vi "Begin (Trap II).vi"(11 "Image Size":T1=enum."160x120") -> (0 "error out":errorcluster)   [LabVIEW 2012]
doc: "Called before other user functions, this VI is expected to open initial I/O refnums, load in file data, and do all program initialization. Notice that the <B>error out</B> terminal is simply used for data flow. Wiring it to other structures or subVIs ensures that this VI runs first."
uses:
  <vilib>/Rock Robotics/WPI/Camera/WPI_CameraImageSize.ctl
  <vilib>/Rock Robotics/WPI/Camera/WPI_CameraWhite Balance Values.ctl
  <vilib>/Rock Robotics/WPI/Camera/WPI_CameraExposure Values.ctl
  <vilib>/Rock Robotics/WPI/Camera/WPI_CameraFrameRate.ctl
  <vilib>/Rock Robotics/WPI/DriverStation/WPI_DriverStationRobotMode2.ctl
  <vilib>/Rock Robotics/WPI/Joystick/WPI_JoystickDeviceEnum.ctl
  <vilib>/Rock Robotics/SystemInterfaces/Typedef/FPGA_TypedefDigitalModule.ctl
  <vilib>/Rock Robotics/SystemInterfaces/DIO/FPGA_DIOPWMChannel.ctl
  <vilib>/Rock Robotics/SystemInterfaces/DIO/FPGA_DIOChannel.ctl
  <vilib>/Rock Robotics/WPI/Encoder/WPI_EncoderType.ctl
  <vilib>/Rock Robotics/WPI/Solenoid/WPI_SolenoidChannel.ctl
  <vilib>/Rock Robotics/SystemInterfaces/Typedef/FPGA_TypedefSolenoidModule.ctl
  <vilib>/Rock Robotics/WPI/Solenoid/WPI_SolenoidValue.ctl
  <vilib>/Rock Robotics/WPI/SafetyOutput/WPI_SafetyOutputConfigMenu.ctl
  <vilib>/Rock Robotics/SystemInterfaces/DIO/FPGA_DIORelayChannel.ctl
  <vilib>/Rock Robotics/SystemInterfaces/Typedef/FPGA_TypedefAnalogModuleForGyro.ctl
  <vilib>/Rock Robotics/SystemInterfaces/AI/FPGA_AIGyroChannel.ctl
  Robot Global Data.vi
  <vilib>/Rock Robotics/WPI/MotorControl/WPI_MotorControlOpen Jaguar.vi
  <vilib>/Rock Robotics/WPI/Counter/WPI_CounterDigitalInputToDigitalSource.vi
  <vilib>/Rock Robotics/WPI/Solenoid/WPI_SolenoidOpenSingle.vi
  <vilib>/Rock Robotics/WPI/Solenoid/WPI_SolenoidSetEnum.vi
  <vilib>/Rock Robotics/WPI/RobotDrive/WPI_RobotDriveOpen2MotorWithJaguar.vi
  <vilib>/Rock Robotics/WPI/Solenoid/WPI_SolenoidOpenDouble.vi
  <vilib>/Rock Robotics/WPI/Compressor/WPI_CompressorGetSetRefNum.vi
  <vilib>/Rock Robotics/WPI/RobotDrive/WPI_RobotDriveOpen4MotorWithTalon.vi
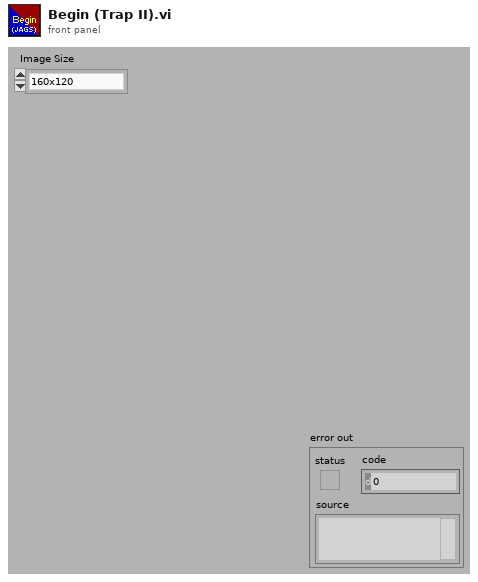
[diagram p1: front panel]
types:
  T1 = typedef "WPI_CameraImageSize.ctl" = enum16{"640x480", "320x240", "160x120"}
  T2 = typedef "FPGA_AIGyroChannel.ctl" = enum8{"AI 1", "AI 2", "Invalid"}
  T3 = typedef "FPGA_TypedefAnalogModuleForGyro.ctl" = enum16{"Analog Module 1"}
  T4 = typedef "WPI_SolenoidChannel.ctl" = enum8{"Solenoid 1", "Solenoid 2", "Solenoid 3", "Solenoid 4", "Solenoid 5", "Solenoid 6", "Solenoid 7", "Solenoid 8", "Invalid"}
  T5 = typedef "WPI_SolenoidValue.ctl" = enum16{"Off", "On", "Forward", "Reverse"}
  T6 = typedef "FPGA_DIOChannel.ctl" = enum8{"DIO 1", "DIO 2", "DIO 3", "DIO 4", "DIO 5", "DIO 6", "DIO 7", "DIO 8", "DIO 9", "DIO 10", "DIO 11", "DIO 12", "DIO 13", "DIO 14", "Invalid"}
  T7 = typedef "FPGA_DIORelayChannel.ctl" = enum8{"Relay 1", "Relay 2", "Relay 3", "Relay 4", "Relay 5", "Relay 6", "Relay 7", "Relay 8", "Invalid"}
  T8 = typedef "FPGA_TypedefDigitalModule.ctl" = enum16{"Digital Module 1", "Digital Module 2"}
  T9 = typedef "WPI_SafetyOutputConfigMenu.ctl" = enum16{"Enable", "Disable"}
  T10 = typedef "FPGA_DIOPWMChannel.ctl" = enum8{"PWM 1", "PWM 2", "PWM 3", "PWM 4", "PWM 5", "PWM 6", "PWM 7", "PWM 8", "PWM 9", "PWM 10", "Invalid"}
  T11 = typedef "WPI_EncoderType.ctl" = enum16{"1x", "2x", "4x"}
  T12 = typedef "FPGA_TypedefSolenoidModule.ctl" = enum16{"Solenoid Module 1", "Solenoid Module 2"}
  T13 = typedef "WPI_JoystickDeviceEnum.ctl" = enum16{"USB 1", "USB 2", "USB 3", "USB 4", "Kinect 1", "Kinect 2"}
  T14 = typedef "WPI_DriverStationRobotMode2.ctl" = enum16{"Autonomous Disabled", "Autonomous Enabled", "Teleop Disabled", "Teleop Enabled", "Timeout", "Finish", "Test Disabled", "Test Enabled"}
  T15 = typedef "WPI_CameraFrameRate.ctl" = u32
  T16 = typedef "WPI_CameraExposure Values.ctl" = enum16{"Auto", "Flicker-free 50 Hz", "Flicker-free 60 Hz", "Hold current"}
  T17 = typedef "WPI_CameraWhite Balance Values.ctl" = enum16{"Auto", "Fixed indoor", "Fixed outdoor 1", "Fixed outdoor 2", "Fixed fluorescent 1", "Fixed fluorescent 2", "Hold current"}
  T18 = typedef "WPI_RobotDriveDevRef.ctl" = cluster{"DevStatus":errorcluster, "Motors[]":T19[], "Square Inputs":bool, "Max Output":dbl, "Isochronous":bool}
  T19 = typedef "WPI_MotorControlDeviceRef.ctl" = cluster{"DeviceStatus":errorcluster, "Type":enum16{"PWM", "CAN"}, "PWM":cluster{"Digital Module":T8, "PWM Channel":T10, "DeadBand":T20}, "CAN":cluster{"Device Number":u8, "Control Mode":T21, "Semaphore":T22, "Max Vout":dbl}, "Invert":bool, "TransformRef":T23, "InvTransformRef":T23}
  T20 = typedef "WPI_PWMDeadband.ctl" = cluster{"Name":string, "maxPositivePwm":i32, "minPositivePwm":i32, "centerPwm":i32, "maxNegativePwm":i32, "minNegativePwm":i32, "angularRange":u16}
  T21 = typedef "WPI_CANJaguar_ControlMode.ctl" = enum8{"Percent VBus", "Current", "Speed", "Position", "Voltage"}
  T22 = typedef "Semaphore RefNum" = refnum<k1>
  T23 = typedef "WPI_PWMTransform_ConPane.ctl" = refnum<vi>
  T24 = typedef "WPI_DigitalInputDevRef.ctl" = cluster{"DevStatus":errorcluster, "DIO Channel":T6, "Digital Module":T8}
  T25 = typedef "FPGA_CounterEncoderSourceConvertionLVSourceType.ctl" = cluster{"DevStatus":errorcluster, "AnalogTriggerMode?":bool, "DigitalMode":cluster{"Digital Module":T8, "DIO Channel":T26}, "AnalogTriggerMode":cluster{"AnalogTriggerIndex":T27, "OutputType":T28}}
  T26 = typedef "FPGA_DIODigitalSourceChannel.ctl" = enum8{"DIO 1", "DIO 2", "DIO 3", "DIO 4", "DIO 5", "DIO 6", "DIO 7", "DIO 8", "DIO 9", "DIO 10", "DIO 11", "DIO 12", "DIO 13", "DIO 14", "Disabled"}
  T27 = typedef "FPGA_AnalogTriggerIndex.ctl" = enum8{"Trig 0", "Trig 1", "Trig 2", "Trig 3", "Trig 4", "Trig 5", "Trig 6", "Trig 7", "Invalid"}
  T28 = typedef "FPGA_AnalogTriggerOutType.ctl" = enum16{"InWindow", "TriggerState", "Rising", "Falling"}
  T29 = typedef "WPI_CameraDevRef.ctl" = cluster{"Camera Address":string, "CameraStatus":errorcluster, "Acquire Image Notifier":refnum<notifier>}
  T30 = typedef "WPI_JoystickDevRef.ctl" = cluster{"Device":T13}
  T31 = typedef "WPI_EncoderDevRef.ctl" = cluster{"DevStatus":errorcluster, "EncoderIndex":T32, "CounterIndex":T33, "DistancePerCount":dbl, "Decoding Type":T11}
  T32 = typedef "FPGA_EncoderIdx.ctl" = enum8{"Enc 0", "Enc 1", "Enc 2", "Enc 3", "Invalid"}
  T33 = typedef "FPGA_CounterCtrSystemIndex.ctl" = enum8{"Ctr 0", "Ctr 1", "Ctr 2", "Ctr 3", "Ctr 4", "Ctr 5", "Ctr 6", "Ctr 7", "Invalid"}
  T34 = typedef "WPI_DigitalOutputDevRef.ctl" = cluster{"Digital Module":T8, "DIO Channel":T6, "DevStatus":errorcluster}
  T35 = typedef "WPI_SolenoidDevRef.ctl" = cluster{"DevStatus":errorcluster, "Solenoid Module":T12, "Forward Solenoid Channel":T4, "Reverse Solenoid Channel":T4}
  T36 = typedef "WPI_GyroDevRef.ctl" = cluster{"DevStatus":errorcluster, "Analog Module":T37, "Analog Channel":T38, "Offset":dbl, "Gain (VoltsPerDegree/Second)":dbl}
  T37 = typedef "FPGA_TypedefAnalogModule.ctl" = enum16{"Analog Module 1", "Analog Module 2"}
  T38 = typedef "FPGA_AIChannel.ctl" = enum8{"AI 1", "AI 2", "AI 3", "AI 4", "AI 5", "AI 6", "AI 7", "AI 8", "Invalid"}
  T39 = typedef "WPI_CompressorDevRef.ctl" = cluster{"DevStatus":errorcluster, "DigitalInputDevRef":T24, "RelayDevRef":T40}
  T40 = typedef "WPI_RelayDevRef.ctl" = cluster{"DevStatus":errorcluster, "Relay Channel":T7, "Digital Module":T8, "Relay Direction":T41}
  T41 = typedef "WPI_RelayDirection.ctl" = enum16{"Both directions", "Forward only", "Reverse only"}
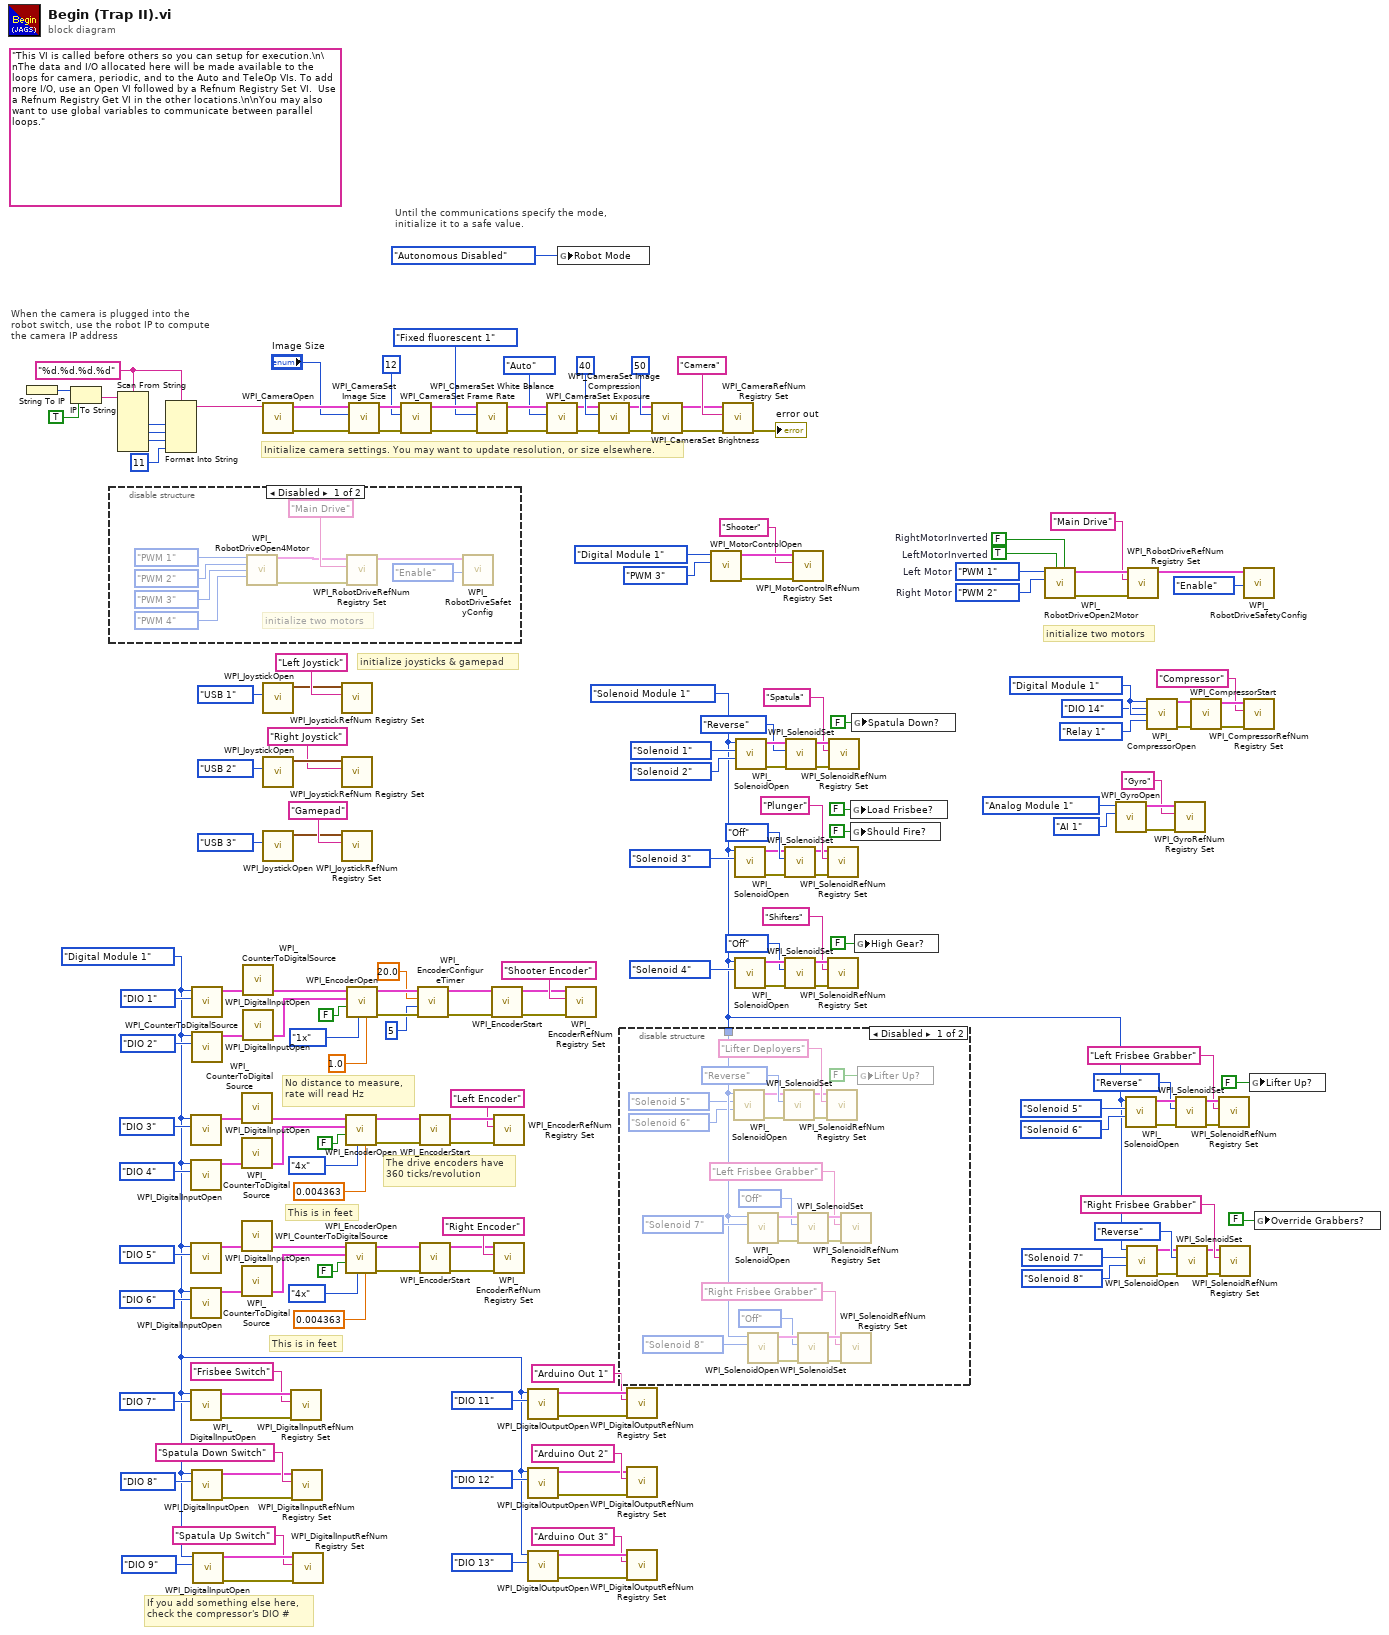
[diagram p0: block diagram]
diagram:
  w53 = FPGA_TypedefDigitalModule."Digital Module 1" ("Pressure Switch Digital Module (Module 1)")
  w77 = FPGA_DIOPWMChannel."PWM 2"  # Right Motor
  w78 = FPGA_DIOPWMChannel."PWM 1"  # Left Motor
  w82 = TRUE  # LeftMotorInverted
  w83 = FALSE  # RightMotorInverted
  w7 = FPGA_TypedefSolenoidModule."Solenoid Module 1" ("Solenoid Module (Module 1)")
  w25 = FPGA_TypedefDigitalModule."Digital Module 1" ("Digital Module (Module 1)")
  w156 = "%d.%d.%d.%d" ("format string")
  (unwired) "This VI is called before others so you can setup for execution.\n\nThe data and I/O allocated here will be made available to the loops for camera, periodic, and to the Auto and TeleOp VIs. To add more I/O, use an Open VI followed by a Refnum Registry Set VI.  Use a Refnum Registry Get VI in the other locations.\n\nYou may also want to use global variables to communicate between parallel loops."
  # "If you add something else here,\ncheck the compressor's DIO #"
  # "No distance to measure,\nrate will read Hz"
  # "The drive encoders have\n360 ticks/revolution"
  # "This is in feet"
  # "This is in feet"
  # "initialize two motors"
  # "initialize joysticks & gamepad"
  # "Until the communications specify the mode,\ninitialize it to a safe value."
  # "When the camera is plugged into the\nrobot switch, use the robot IP to compute\nthe camera IP address"
  # "Initialize camera settings. You may want to update resolution, or size elsewhere."
  n1 = String To IP() -> (0:w163:u32)  [unwired: 1 in]
  n2 = IP To String(1:TRUE ("dot notation? (F)"), 2:w163) -> (0:w161:string)
  n3 = disable-structure shown="Disabled" {
    frame Disabled {
      # "initialize two motors"
      n4 = call-poly <vilib>:"WPI_RobotDriveOpen4Motor.vi"("Rear Left Motor"=FPGA_DIOPWMChannel."PWM 1", "Rear Right Motor"=FPGA_DIOPWMChannel."PWM 2" ("Rear Left Motor"), "Front Left Motor"=FPGA_DIOPWMChannel."PWM 3" ("Rear Left Motor"), "Front Right Motor"=FPGA_DIOPWMChannel."PWM 4" ("Rear Left Motor")) -> ("RobotDriveDevRef"=w190:T18, "error out"=w189:errorcluster)  [unwired: 10 in]
      n5 = call <vilib>:"WPI_RobotDriveRefNum Registry Set.vi"("error in (no error)"=w189, "refnum name"="Main Drive", "RobotDriveDevRef"=w190) -> ("RobotDriveDevRef"=w192:T18)  [unwired: 8 out]
      n6 = call <vilib>:"WPI_RobotDriveSafetyConfig.vi"("mode"=WPI_SafetyOutputConfigMenu."Enable", "RobotDriveDevRef"=w192) -> ()  [unwired: 8 in, 2 out]
    }
    frame Enabled {
    }
  }
  n7 = Scan From String(format string=w156, input string=w161) -> (output 1=w160:i32, output 2=w159:i32, output 3=w158:i32)  [unwired: 7 in, 3 out]
  n8 = Format Into String(format string=w156, w160, w159, w158, 11 ("Compression")) -> (resulting string=w154:string)  [unwired: 2 in, 1 out]
  n9 = call <vilib>:"WPI_DigitalInputOpen.vi"("DIO Channel"=FPGA_DIOChannel."DIO 3" ("CS Channel"), "Digital Module (Module 1)"=w25) -> ("DigitalInputDevRef"=w105:T24)  [unwired: 1 in, 8 out]
  n10 = call <vilib>:"WPI_DigitalInputOpen.vi"("DIO Channel"=FPGA_DIOChannel."DIO 4" ("Clock Channel"), "Digital Module (Module 1)"=w25) -> ("DigitalInputDevRef"=w106:T24)  [unwired: 1 in, 8 out]
  n11 = call <vilib>:"WPI_DigitalInputOpen.vi"("DIO Channel"=FPGA_DIOChannel."DIO 5" ("CS Channel"), "Digital Module (Module 1)"=w25) -> ("DigitalInputDevRef"=w90:T24)  [unwired: 1 in, 8 out]
  n12 = call <vilib>:"WPI_DigitalInputOpen.vi"("DIO Channel"=FPGA_DIOChannel."DIO 6" ("Clock Channel"), "Digital Module (Module 1)"=w25) -> ("DigitalInputDevRef"=w89:T24)  [unwired: 1 in, 8 out]
  n13 = call <vilib>:"WPI_DigitalInputOpen.vi"("DIO Channel"=FPGA_DIOChannel."DIO 7", "Digital Module (Module 1)"=w25) -> ("error out"=w55:errorcluster, "DigitalInputDevRef"=w56:T24)  [unwired: 8 in]
  n14 = call <vilib>:"WPI_DigitalInputOpen.vi"("DIO Channel"=FPGA_DIOChannel."DIO 1" ("CS Channel"), "Digital Module (Module 1)"=w25) -> ("DigitalInputDevRef"=w131:T24)  [unwired: 1 in, 8 out]
  n15 = call <vilib>:"WPI_DigitalInputOpen.vi"("DIO Channel"=FPGA_DIOChannel."DIO 2" ("Clock Channel"), "Digital Module (Module 1)"=w25) -> ("DigitalInputDevRef"=w130:T24)  [unwired: 1 in, 8 out]
  n16 = call <vilib>:"WPI_DigitalInputOpen.vi"("DIO Channel"=FPGA_DIOChannel."DIO 8", "Digital Module (Module 1)"=w25) -> ("error out"=w44:errorcluster, "DigitalInputDevRef"=w43:T24)  [unwired: 8 in]
  n17 = call <vilib>:"WPI_DigitalInputOpen.vi"("DIO Channel"=FPGA_DIOChannel."DIO 9", "Digital Module (Module 1)"=w25) -> ("error out"=w39:errorcluster, "DigitalInputDevRef"=w40:T24)  [unwired: 8 in]
  n18 = call-poly <vilib>:"WPI_CounterToDigitalSource.vi"("DigitalInputDevRef"=w105) -> ("Digital Source"=w102:T25)  [unwired: 6 out]
  n19 = call-poly <vilib>:"WPI_CounterToDigitalSource.vi"("DigitalInputDevRef"=w106) -> ("Digital Source"=w103:T25)  [unwired: 6 out]
  n20 = call-poly <vilib>:"WPI_CounterToDigitalSource.vi"("DigitalInputDevRef"=w90) -> ("Digital Source"=w93:T25)  [unwired: 6 out]
  n21 = call-poly <vilib>:"WPI_CounterToDigitalSource.vi"("DigitalInputDevRef"=w89) -> ("Digital Source"=w92:T25)  [unwired: 6 out]
  n22 = call-poly <vilib>:"WPI_CounterToDigitalSource.vi"("DigitalInputDevRef"=w131) -> ("Digital Source"=w134:T25)  [unwired: 6 out]
  n23 = call-poly <vilib>:"WPI_CounterToDigitalSource.vi"("DigitalInputDevRef"=w130) -> ("Digital Source"=w133:T25)  [unwired: 6 out]
  n24 = call <vilib>:"WPI_CameraOpen.vi"("Camera Address"=w154) -> ("error out"=w175:errorcluster, "CameraDevRef"=w176:T29)  [unwired: 1 in, 8 out]
  n25 = call <vilib>:"WPI_JoystickOpen.vi"("JoystickDevice"=WPI_JoystickDeviceEnum."USB 1") -> ("JoystickDevRef"=w152:T30)  [unwired: 10 in]
  n26 = call <vilib>:"WPI_JoystickOpen.vi"("JoystickDevice"=WPI_JoystickDeviceEnum."USB 2") -> ("JoystickDevRef"=w148:T30)  [unwired: 10 in]
  n27 = call <vilib>:"WPI_JoystickOpen.vi"("JoystickDevice"=WPI_JoystickDeviceEnum."USB 3") -> ("JoystickDevRef"=w145:T30)  [unwired: 10 in]
  n28 = call <vilib>:"WPI_DigitalInputRefNum Registry Set.vi"("error in (no error)"=w55, "refnum name"="Frisbee Switch", "DigitalInputDevRef"=w56) -> ()  [unwired: 7 in, 2 out]
  n29 = call <vilib>:"WPI_DigitalInputRefNum Registry Set.vi"("error in (no error)"=w44, "refnum name"="Spatula Down Switch", "DigitalInputDevRef"=w43) -> ()  [unwired: 7 in, 2 out]
  n30 = call <vilib>:"WPI_DigitalInputRefNum Registry Set.vi"("error in (no error)"=w39, "refnum name"="Spatula Up Switch", "DigitalInputDevRef"=w40) -> ()  [unwired: 7 in, 2 out]
  n31 = call <vilib>:"WPI_JoystickRefNum Registry Set.vi"("refnum name"="Left Joystick", "JoystickDevRef"=w152) -> ()  [unwired: 8 in, 2 out]
  n32 = call <vilib>:"WPI_JoystickRefNum Registry Set.vi"("refnum name"="Right Joystick", "JoystickDevRef"=w148) -> ()  [unwired: 8 in, 2 out]
  n33 = call <vilib>:"WPI_JoystickRefNum Registry Set.vi"("refnum name"="Gamepad", "JoystickDevRef"=w145) -> ()  [unwired: 8 in, 2 out]
  n34 = call <vilib>:"WPI_EncoderOpen.vi"("DistancePerCount"=0.004363, "Decoding Type"=WPI_EncoderType."4x", "Invert Direction (False)"=FALSE, "BSource"=w103, "ASource"=w102) -> ("error out"=w108:errorcluster, "EncoderDevRef"=w107:T31)  [unwired: 5 in]
  n35 = call <vilib>:"WPI_EncoderOpen.vi"("DistancePerCount"=0.004363, "Decoding Type"=WPI_EncoderType."4x", "Invert Direction (False)"=FALSE, "BSource"=w92, "ASource"=w93) -> ("error out"=w87:errorcluster, "EncoderDevRef"=w88:T31)  [unwired: 5 in]
  n36 = call <vilib>:"WPI_EncoderOpen.vi"("DistancePerCount"=1.0, "Decoding Type"=WPI_EncoderType."1x", "Invert Direction (False)"=FALSE, "BSource"=w133, "ASource"=w134) -> ("error out"=w63:errorcluster, "EncoderDevRef"=w64:T31)  [unwired: 5 in]
  n37 = call <vilib>:"WPI_CameraSet Image Size.vi"("error in (no error)"=w175, "Image Size"="Image Size", "CameraDevRef"=w176) -> ("error out"=w174:errorcluster, "CameraDevRef Out"=w177:T29)  [unwired: 7 out]
  n38 = call <vilib>:"WPI_CameraSet Frame Rate.vi"("error in (no error)"=w174, "Frame Rate (fps)"=T15 12, "CameraDevRef"=w177) -> ("error out"=w173:errorcluster, "CameraDevRef Out"=w179:T29)  [unwired: 7 out]
  n39 = call <vilib>:"WPI_EncoderConfigureTimer.vi"("error in (no error)"=w63, "Number Samples to Average"=u8 5, "Minimum Rate"=20.0, "EncoderDevRef"=w64) -> ("error out"=w62:errorcluster, "EncoderDevRef"=w61:T31)  [unwired: 6 in]
  n40 = call <vilib>:"WPI_EncoderStart.vi"("error in (no error)"=w108, "EncoderDevRef"=w107) -> ("error out"=w109:errorcluster, "EncoderDevRef"=w110:T31)  [unwired: 8 in]
  n41 = call <vilib>:"WPI_EncoderStart.vi"("error in (no error)"=w87, "EncoderDevRef"=w88) -> ("error out"=w86:errorcluster, "EncoderDevRef"=w85:T31)  [unwired: 8 in]
  n42 = call <vilib>:"WPI_CameraSet White Balance.vi"("error in (no error)"=w173, "White Balance"=WPI_CameraWhite_Balance_Values."Fixed fluorescent 1", "CameraDevRef"=w179) -> ("error out"=w172:errorcluster, "CameraDevRef Out"=w178:T29)  [unwired: 7 out]
  n43 = call <vilib>:"WPI_EncoderStart.vi"("error in (no error)"=w62, "EncoderDevRef"=w61) -> ("error out"=w129:errorcluster, "EncoderDevRef"=w128:T31)  [unwired: 8 in]
  n44 = call <vilib>:"WPI_EncoderRefNum Registry Set.vi"("error in (no error)"=w109, "refnum name"="Left Encoder", "EncoderDevRef"=w110) -> ()  [unwired: 7 in, 2 out]
  n45 = call <vilib>:"WPI_EncoderRefNum Registry Set.vi"("error in (no error)"=w86, "refnum name"="Right Encoder", "EncoderDevRef"=w85) -> ()  [unwired: 7 in, 2 out]
  n46 = call <vilib>:"WPI_DigitalOutputOpen.vi"("DIO Channel"=FPGA_DIOChannel."DIO 11", "Digital Module (Module 1)"=w25) -> ("error out"=w35:errorcluster, "DigitalOutputDevRef"=w36:T34)  [unwired: 8 in]
  n47 = call <vilib>:"WPI_DigitalOutputOpen.vi"("DIO Channel"=FPGA_DIOChannel."DIO 12", "Digital Module (Module 1)"=w25) -> ("error out"=w32:errorcluster, "DigitalOutputDevRef"=w31:T34)  [unwired: 8 in]
  n48 = call <vilib>:"WPI_DigitalOutputOpen.vi"("DIO Channel"=FPGA_DIOChannel."DIO 13", "Digital Module (Module 1)"=w25) -> ("error out"=w27:errorcluster, "DigitalOutputDevRef"=w28:T34)  [unwired: 8 in]
  n49 = call <vilib>:"WPI_CameraSet Exposure.vi"("error in (no error)"=w172, "Exposure"=WPI_CameraExposure_Values."Auto", "CameraDevRef"=w178) -> ("error out"=w171:errorcluster, "CameraDevRef Out"=w181:T29)  [unwired: 7 out]
  n50 = global write "Robot Global Data.vi" "Robot Mode"(WPI_DriverStationRobotMode2."Autonomous Disabled" ("Robot Mode")) -> ()
  n51 = call <vilib>:"WPI_EncoderRefNum Registry Set.vi"("error in (no error)"=w129, "refnum name"="Shooter Encoder", "EncoderDevRef"=w128) -> ()  [unwired: 7 in, 2 out]
  n52 = call <vilib>:"WPI_CameraSet Image Compression.vi"("error in (no error)"=w171, "Compression"=40, "CameraDevRef"=w181) -> ("error out"=w170:errorcluster, "CameraDevRef Out"=w180:T29)  [unwired: 7 out]
  n53 = disable-structure shown="Disabled" {
    disable-tunnel: w7 -> [w205 _]
    frame Disabled {
      n54 = call-poly <vilib>:"WPI_SolenoidOpen.vi"("Reverse Solenoid Channel"=WPI_SolenoidChannel."Solenoid 6", "Forward Solenoid Channel"=WPI_SolenoidChannel."Solenoid 5" ("Solenoid Channel"), "Solenoid Module (Module 1)"=w205) -> ("error out"=w198:errorcluster, "SolenoidDevRef"=w197:T35)  [unwired: 7 in]
      n55 = call-poly <vilib>:"WPI_SolenoidOpen.vi"("Solenoid Channel"=WPI_SolenoidChannel."Solenoid 7", "Solenoid Module (Module 1)"=w205) -> ("error out"=w215:errorcluster, "SolenoidDevRef"=w214:T35)  [unwired: 8 in]
      n56 = call-poly <vilib>:"WPI_SolenoidOpen.vi"("Solenoid Channel"=WPI_SolenoidChannel."Solenoid 8", "Solenoid Module (Module 1)"=w205) -> ("error out"=w210:errorcluster, "SolenoidDevRef"=w211:T35)  [unwired: 8 in]
      n57 = call-poly <vilib>:"WPI_SolenoidSet.vi"("error in (no error)"=w198, "Value"=WPI_SolenoidValue."Reverse", "SolenoidDevRef"=w197) -> ("error out"=w199:errorcluster, "SolenoidDevRef"=w200:T35)  [unwired: 7 in]
      n58 = call-poly <vilib>:"WPI_SolenoidSet.vi"("error in (no error)"=w215, "Value"=WPI_SolenoidValue."Off", "SolenoidDevRef"=w214) -> ("error out"=w216:errorcluster, "SolenoidDevRef"=w217:T35)  [unwired: 7 in]
      n59 = call-poly <vilib>:"WPI_SolenoidSet.vi"("error in (no error)"=w210, "Value"=WPI_SolenoidValue."Off", "SolenoidDevRef"=w211) -> ("error out"=w209:errorcluster, "SolenoidDevRef"=w208:T35)  [unwired: 7 in]
      n60 = call <vilib>:"WPI_SolenoidRefNum Registry Set.vi"("error in (no error)"=w199, "refnum name"="Lifter Deployers", "SolenoidDevRef"=w200) -> ()  [unwired: 7 in, 2 out]
      n61 = call <vilib>:"WPI_SolenoidRefNum Registry Set.vi"("error in (no error)"=w216, "refnum name"="Left Frisbee Grabber", "SolenoidDevRef"=w217) -> ()  [unwired: 7 in, 2 out]
      n62 = call <vilib>:"WPI_SolenoidRefNum Registry Set.vi"("error in (no error)"=w209, "refnum name"="Right Frisbee Grabber", "SolenoidDevRef"=w208) -> ()  [unwired: 7 in, 2 out]
      n63 = global write "Robot Global Data.vi" "Lifter Up?"(FALSE ("High Gear?")) -> ()
    }
    frame Enabled {
    }
  }
  n64 = call <vilib>:"WPI_DigitalOutputRefNum Registry Set.vi"("error in (no error)"=w35, "refnum name"="Arduino Out 1", "DigitalOutputDevRef"=w36) -> ()  [unwired: 7 in, 2 out]
  n65 = call <vilib>:"WPI_DigitalOutputRefNum Registry Set.vi"("error in (no error)"=w32, "refnum name"="Arduino Out 2", "DigitalOutputDevRef"=w31) -> ()  [unwired: 7 in, 2 out]
  n66 = call <vilib>:"WPI_DigitalOutputRefNum Registry Set.vi"("error in (no error)"=w27, "refnum name"="Arduino Out 3", "DigitalOutputDevRef"=w28) -> ()  [unwired: 7 in, 2 out]
  n67 = call <vilib>:"WPI_CameraSet Brightness.vi"("error in (no error)"=w170, "Brightness"=50, "CameraDevRef"=w180) -> ("error out"=w168:errorcluster, "CameraDevRef Out"=w169:T29)  [unwired: 7 out]
  n68 = call-poly <vilib>:"WPI_MotorControlOpen.vi"("PWM Channel"=FPGA_DIOPWMChannel."PWM 3", "Digital Module (Module 1)"=FPGA_TypedefDigitalModule."Digital Module 1") -> ("error out"=w140:errorcluster, "MotorControlDeviceRef"=w141:T19)  [unwired: 8 in]
  n69 = call <vilib>:"WPI_CameraRefNum Registry Set.vi"("error in (no error)"=w168, "refnum name"="Camera", "CameraDevRef"=w169) -> ("error out"=→"error out":errorcluster)  [unwired: 8 out]
  n70 = call-poly <vilib>:"WPI_SolenoidOpen.vi"("Solenoid Channel"=WPI_SolenoidChannel."Solenoid 3", "Solenoid Module (Module 1)"=w7) -> ("error out"=w117:errorcluster, "SolenoidDevRef"=w116:T35)  [unwired: 8 in]
  n71 = call-poly <vilib>:"WPI_SolenoidOpen.vi"("Solenoid Channel"=WPI_SolenoidChannel."Solenoid 4", "Solenoid Module (Module 1)"=w7) -> ("error out"=w71:errorcluster, "SolenoidDevRef"=w72:T35)  [unwired: 8 in]
  n72 = call-poly <vilib>:"WPI_SolenoidOpen.vi"("Reverse Solenoid Channel"=WPI_SolenoidChannel."Solenoid 2", "Forward Solenoid Channel"=WPI_SolenoidChannel."Solenoid 1" ("Solenoid Channel"), "Solenoid Module (Module 1)"=w7) -> ("error out"=w125:errorcluster, "SolenoidDevRef"=w126:T35)  [unwired: 7 in]
  n73 = call-poly <vilib>:"WPI_SolenoidSet.vi"("error in (no error)"=w117, "Value"=WPI_SolenoidValue."Off", "SolenoidDevRef"=w116) -> ("error out"=w118:errorcluster, "SolenoidDevRef"=w119:T35)  [unwired: 7 in]
  n74 = call-poly <vilib>:"WPI_SolenoidSet.vi"("error in (no error)"=w71, "Value"=WPI_SolenoidValue."Off", "SolenoidDevRef"=w72) -> ("error out"=w70:errorcluster, "SolenoidDevRef"=w69:T35)  [unwired: 7 in]
  n75 = call-poly <vilib>:"WPI_SolenoidSet.vi"("error in (no error)"=w125, "Value"=WPI_SolenoidValue."Reverse", "SolenoidDevRef"=w126) -> ("error out"=w124:errorcluster, "SolenoidDevRef"=w123:T35)  [unwired: 7 in]
  n76 = call <vilib>:"WPI_MotorControlRefNum Registry Set.vi"("error in (no error)"=w140, "refnum name"="Shooter", "MotorControlDevRef"=w141) -> ()  [unwired: 7 in, 2 out]
  n77 = call <vilib>:"WPI_SolenoidRefNum Registry Set.vi"("error in (no error)"=w118, "refnum name"="Plunger", "SolenoidDevRef"=w119) -> ()  [unwired: 7 in, 2 out]
  n78 = call <vilib>:"WPI_SolenoidRefNum Registry Set.vi"("error in (no error)"=w70, "refnum name"="Shifters", "SolenoidDevRef"=w69) -> ()  [unwired: 7 in, 2 out]
  n79 = call <vilib>:"WPI_SolenoidRefNum Registry Set.vi"("error in (no error)"=w124, "refnum name"="Spatula", "SolenoidDevRef"=w123) -> ()  [unwired: 7 in, 2 out]
  n80 = global write "Robot Global Data.vi" "Load Frisbee?"(FALSE ("High Gear?")) -> ()
  n81 = global write "Robot Global Data.vi" "Should Fire?"(FALSE ("High Gear?")) -> ()
  n82 = global write "Robot Global Data.vi" "Spatula Down?"(FALSE ("High Gear?")) -> ()
  n83 = global write "Robot Global Data.vi" "High Gear?"(FALSE ("High Gear?")) -> ()
  n84 = call-poly <vilib>:"WPI_RobotDriveOpen2Motor.vi"("Right Motor Inverted"=w83, "Left Motor Inverted"=w82, "Right Motor"=w77, "Left Motor"=w78) -> ("error out"=w79:errorcluster, "RobotDriveDevRef"=w81:T18)  [unwired: 1 in, 5 out]
  n85 = call <vilib>:"WPI_GyroOpen.vi"("Analog Channel"=FPGA_AIGyroChannel."AI 1", "Analog Module (Module 1)"=FPGA_TypedefAnalogModuleForGyro."Analog Module 1") -> ("error out"=w5:errorcluster, "GyroDevRef"=w4:T36)  [unwired: 7 in, 1 out]
  n86 = call-poly <vilib>:"WPI_SolenoidOpen.vi"("Reverse Solenoid Channel"=WPI_SolenoidChannel."Solenoid 6", "Forward Solenoid Channel"=WPI_SolenoidChannel."Solenoid 5" ("Solenoid Channel"), "Solenoid Module (Module 1)"=w7) -> ("error out"=w20:errorcluster, "SolenoidDevRef"=w21:T35)  [unwired: 7 in]
  n87 = call-poly <vilib>:"WPI_SolenoidOpen.vi"("Reverse Solenoid Channel"=WPI_SolenoidChannel."Solenoid 8", "Forward Solenoid Channel"=WPI_SolenoidChannel."Solenoid 7" ("Solenoid Channel"), "Solenoid Module (Module 1)"=w7) -> ("error out"=w11:errorcluster, "SolenoidDevRef"=w10:T35)  [unwired: 7 in]
  n88 = call <vilib>:"WPI_RobotDriveRefNum Registry Set.vi"("error in (no error)"=w79, "refnum name"="Main Drive", "RobotDriveDevRef"=w81) -> ("RobotDriveDevRef"=w76:T18)  [unwired: 8 out]
  n89 = call <vilib>:"WPI_CompressorOpen.vi"("Pressure Switch Digital Module (Module 1)"=w53, "Pressure Switch DIO Channel"=FPGA_DIOChannel."DIO 14", "Relay Digital Module (Module 1)"=w53, "Relay Channel"=FPGA_DIORelayChannel."Relay 1") -> ("CompressorDevRef"=w49:T39, "error out"=w50:errorcluster)  [unwired: 10 in]
  n90 = call <vilib>:"WPI_GyroRefNum Registry Set.vi"("error in (no error)"=w5, "refnum name"="Gyro", "GyroDevRef"=w4) -> ()  [unwired: 7 in, 2 out]
  n91 = call-poly <vilib>:"WPI_SolenoidSet.vi"("error in (no error)"=w20, "Value"=WPI_SolenoidValue."Reverse", "SolenoidDevRef"=w21) -> ("error out"=w19:errorcluster, "SolenoidDevRef"=w18:T35)  [unwired: 7 in]
  n92 = call-poly <vilib>:"WPI_SolenoidSet.vi"("error in (no error)"=w11, "Value"=WPI_SolenoidValue."Reverse", "SolenoidDevRef"=w10) -> ("error out"=w12:errorcluster, "SolenoidDevRef"=w13:T35)  [unwired: 7 in]
  n93 = call <vilib>:"WPI_CompressorStart.vi"("error in (no error)"=w50, "CompressorDevRef"=w49) -> ("error out"=w48:errorcluster, "CompressorDevRef"=w47:T39)  [unwired: 8 in]
  n94 = call <vilib>:"WPI_SolenoidRefNum Registry Set.vi"("error in (no error)"=w19, "refnum name"="Left Frisbee Grabber", "SolenoidDevRef"=w18) -> ()  [unwired: 7 in, 2 out]
  n95 = call <vilib>:"WPI_SolenoidRefNum Registry Set.vi"("error in (no error)"=w12, "refnum name"="Right Frisbee Grabber", "SolenoidDevRef"=w13) -> ()  [unwired: 7 in, 2 out]
  n96 = call <vilib>:"WPI_RobotDriveSafetyConfig.vi"("mode"=WPI_SafetyOutputConfigMenu."Enable", "RobotDriveDevRef"=w76) -> ()  [unwired: 8 in, 2 out]
  n97 = call <vilib>:"WPI_CompressorRefNum Registry Set.vi"("error in (no error)"=w48, "refnum name"="Compressor", "CompressorDevRef"=w47) -> ()  [unwired: 7 in, 2 out]
  n98 = global write "Robot Global Data.vi" "Lifter Up?"(FALSE ("High Gear?")) -> ()
  n99 = global write "Robot Global Data.vi" "Override Grabbers?"(FALSE ("High Gear?")) -> ()
